vi "LVPortBindPropertyToControl.vi"(0 "pID":string, 5 "Control To Bind":refnum<vi>, 7 "Controls To Bind":refnum<vi>[](array[refnum]), 9 "Direction":T1) -> (4 "pID out":string)   [LabVIEW 2017]
uses:
  LVPortControlBindingDirectionEnum.ctl
  <userlib>/_OpenG.lib/dictionary/dictionary.llb/Dictionary Key Value Pair Cluster__ogtk.ctl
  LVPortControlBindingInfoType.ctl
  <userlib>/_OpenG.lib/dictionary/dictionary.llb/Dictionary Update (by scalar value)__ogtk.vi
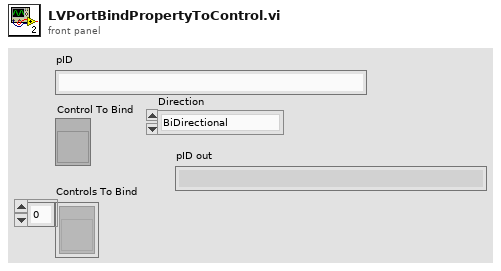
[diagram p1: front panel]
types:
  T1 = typedef "LVPortControlBindingDirectionEnum.ctl" = enum16{"BiDirectional", "ToMatlab", "ToLabview"}
  T2 = typedef "Dictionary Object RefNum__ogtk.ctl" = refnum<k1>
  T3 = typedef "LVPortControlBindingInfoType.ctl" = cluster{"Bound Control":refnum<vi>, "Name":string, "Direction":T1, "Event Register":refnum<event-registration>}
  T4 = typedef "Dictionary Key Value Pair Cluster__ogtk.ctl" = cluster{"key":variant, "value":variant}
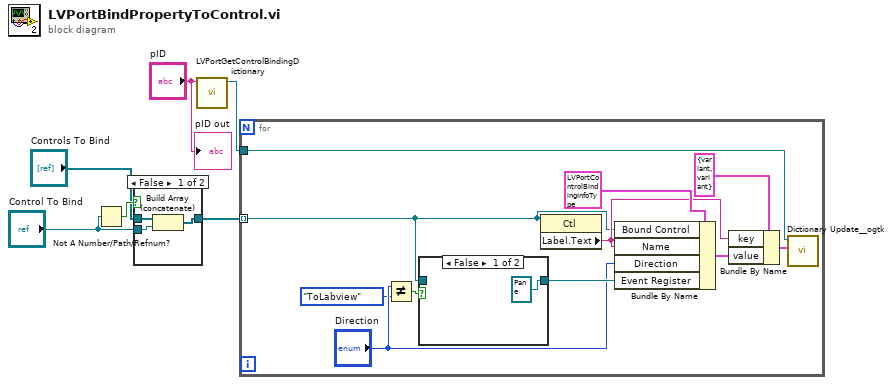
[diagram p0: block diagram]
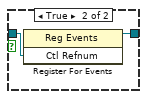
[diagram p2: hidden frame]
diagram:
  n1 = Not A Number/Path/Refnum?(number/path/refnum="Control To Bind") -> (NaN/Path/Refnum?=w6:bool)
  n2 = case shown="False" w6 {
    tunnel: "Controls To Bind" -> [w9 w10]
    tunnel: "Control To Bind" -> [w8 _]
    tunnel: [w7 w10] -> w2
    frame False {
      n3 = Build Array (concatenate)(w9, w8) -> (w7:refnum<vi>[])
    }
    frame True {
    }
  }
  n4 = call "LVPortGetControlBindingDictionary.vi"("pID"="pID") -> ("Refnum out"=w1:T2)  [unwired: 10 in]
  n5 = for {
    tunnel: w2 -> [w15] mode=indexing
    tunnel: w1 -> [w19]
    n6 = Not Equal?(x="Direction", y=LVPortControlBindingDirectionEnum."ToLabview") -> (x != y?=w11:bool)
    n7 = case shown="False" w11 {
      tunnel: w15 -> [_ w24]
      tunnel: [refnum<event-registration> refnum ("Event Registration Refnum") w23] -> w14
      frame False {
      }
      frame True {
        n8 = register-events(w24) -> (reference out=w23:refnum<event-registration>)  [unwired: 2 in, 1 out]
      }
    }
    n9 = property class="Ctl"(reference=w15) -> ("Label.Text"=w17:string)  [unwired: 1 in, 2 out]
    n10 = Bundle By Name(cluster=T3 {"Bound Control"=refnum, "Name"="", "Direction"=enum."BiDirectional", "Event Register"=refnum}, "Bound Control"=w15, "Name"=w17, "Direction"="Direction", "Event Register"=w14) -> (w16:T3)
    n11 = Bundle By Name(cluster=T4 {"key"=variant, "value"=variant} ("key-value"), "key"=w17, "value"=w16) -> (w20:T4)
    n12 = call-poly <userlib>:"Dictionary Update__ogtk.vi"("key-value"=w20, "dictionary"=w19) -> ()  [unwired: 7 in, 3 out]
  }
  "pID out" <- "pID"
